vi "initialise.vi"(8 "error in (no error)":errorcluster, 11 "DL090623TwoDAnalyser in":refnum<class "AnalyserDL090623TwoD.lvclass">) -> (0 "error out":errorcluster, 3 "DL090623TwoDAnalyser out":refnum<class "AnalyserDL090623TwoD.lvclass">)   [LabVIEW 2010, in "AnalyserDL090623TwoD.lvclass"]
doc: "The dynamic dispatch-version of this VI initalises the plug-in object by allocating and initalising any dynamic resources need."
uses:
  AnalyserDL090623TwoD.lvclass
  common/classes/Image/Image/Image.lvclass
  AnalyserDL090624Scaffold/AnalyserDL090624Scaffold/AnalyserDL090624Scaffold.lvclass
  Segmenter/GenericSegmenter/GenericSegmenter/GenericSegmenter.lvclass
  TraceProcessor/GenericTraceProcessor/GenericTraceProcessor/GenericTraceProcessor.lvclass
  common/classes/ErrorController/ErrorController/ErrorController.lvclass
  common/enumerations/top-level_component_type_enum.ctl
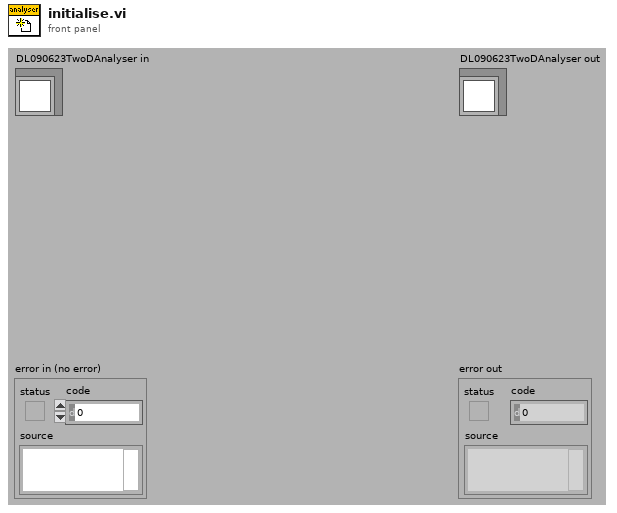
[diagram p1: front panel]
types:
  T1 = typedef "top-level_component_type_enum.ctl" = enum16{"undefined", "ImagingMode", "ScanHead", "DAQ", "ImageAssembler", "Display", "DataCollection", "Analyser", "Stimulator", "ExperimentController", "Instrument", "Stage"}
  T2 = typedef "Image Type" = u32
  T3 = typedef "plugin_specification.ctl" = cluster{"class path":string, "configuration":string, "label":string, "settings name":string}
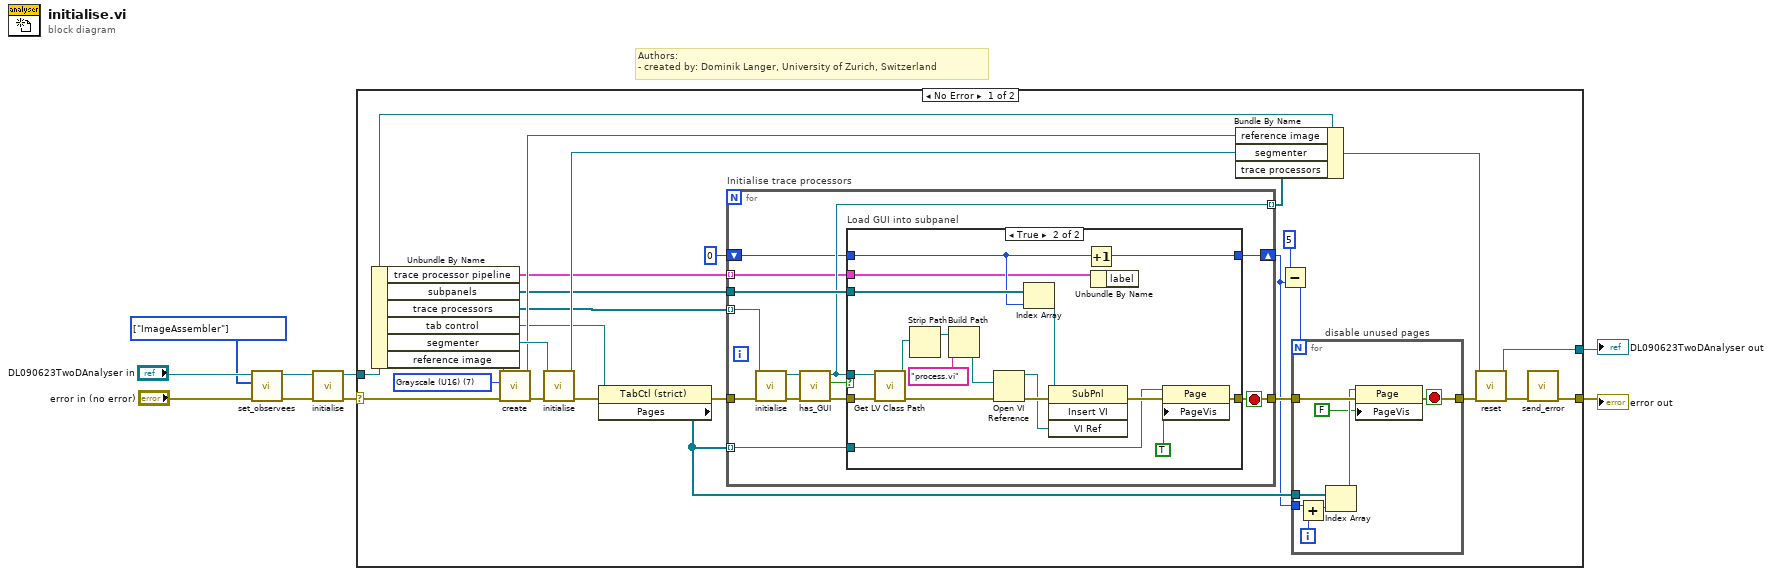
[diagram p0: block diagram]
diagram:
  w1 = T1[] [enum."ImageAssembler"] items=["undefined", "ImagingMode", "ScanHead", "DAQ", "ImageAssembler", "Display", "DataCollection", "Analyser", "Stimulator", "ExperimentController", "Instrument", "Stage"] ("observees")
  # "Authors: \n- created by: Dominik Langer, University of Zurich, Switzerland"
  n1 = call-dynamic "set_observees.vi"("error in (no error)"="error in (no error)", "observees"=w1, "GenericToplevelComponent in"="DL090623TwoDAnalyser in") -> ("error out"=w2:errorcluster, "GenericToplevelComponent out"=w4:refnum<class "AnalyserDL090623TwoD.lvclass">)  [unwired: 7 in]
  n2 = call-parent "initialise.vi"("error in (no error)"=w2, "GenericPlugin in"=w4) -> ("error out"=w9:errorcluster, "GenericPlugin out"=w8:refnum<class "AnalyserDL090623TwoD.lvclass">)  [unwired: 8 out]
  n3 = case shown="No Error" w9 {
    selector: w9 -> [w10 w78]
    tunnel: w8 -> [w11 w77]
    tunnel: [w12 w78] -> w7
    tunnel: [w32 w77] -> w6
    frame No Error {
      w34 = T2 7 items=["Grayscale (U8)", "Grayscale (I16)", "Grayscale (SGL)", "Complex (CSG)", "RGB (U32)", "HSL (U32)", "RGB (U64)", "Grayscale (U16)"] ("Image Type")
      n4 = Unbundle By Name(w11) -> ("trace processor pipeline"=w20:T3[], "subpanels"=w25:refnum<vi>[], "trace processors"=w27:refnum<class "GenericTraceProcessor.lvclass">[], "tab control"=w21:refnum<vi>, "segmenter"=w31:refnum<class "GenericSegmenter.lvclass">, "reference image"=w35:refnum<class "Image.lvclass">)
      n5 = call "create.vi"("error in (no error)"=w10, "Image Type"=w34, "Image in"=w35) -> ("error out"=w30:errorcluster, "Image out"=w28:refnum<class "Image.lvclass">)  [unwired: 1 in, 6 out]
      n6 = call-dynamic "initialise.vi"("error in (no error)"=w30, "GenericPlugin in"=w31) -> ("error out"=w23:errorcluster, "GenericPlugin out"=w29:refnum<class "GenericSegmenter.lvclass">)  [unwired: 8 out]
      n7 = property class="TabCtl (strict)"(reference=w21, error in=w23) -> (error out=w22:errorcluster, "Pages"=w17:refnum<vi>[])  [unwired: 1 out]
      n8 = for "Initialise trace processors" {
        tunnel: w27 -> [w55] mode=indexing
        tunnel: [w49] -> w26 mode=indexing
        tunnel: w25 -> [w51]
        shift-right: [w47] -> w16
        shift-left: 0 -> [w48]
        tunnel: w17 -> [w46] mode=indexing
        tunnel: w20 -> [w45] mode=indexing
        tunnel: w22 -> [w56]
        tunnel: [w44] -> w19
        stop <- w44 stop-if-true
        n9 = call-dynamic "initialise.vi"("error in (no error)"=w56, "GenericPlugin in"=w55) -> ("error out"=w54:errorcluster, "GenericPlugin out"=w53:refnum<class "GenericTraceProcessor.lvclass">)  [unwired: 8 out]
        n10 = call-dynamic "has_GUI.vi"("error in (no error)"=w54, "GenericTraceProcessor in"=w53) -> ("error out"=w52:errorcluster, "has GUI?"=w50:bool, "GenericTraceProcessor out"=w49:refnum<class "GenericTraceProcessor.lvclass">)  [unwired: 7 out]
        n11 = case "Load GUI into subpanel" shown="True" w50 {
          tunnel: w52 -> [w58 w72]
          tunnel: [w58 w62] -> w44
          tunnel: w51 -> [_ w76]
          tunnel: w49 -> [_ w70]
          tunnel: w48 -> [w57 w64]
          tunnel: [w57 w65] -> w47
          tunnel: w46 -> [_ w61]
          tunnel: w45 -> [_ w60]
          frame False {
          }
          frame True {
            n12 = call <vilib>:"Get LV Class Path.vi"("error in (no error)"=w72, "object"=w70) -> ("error out"=w71:errorcluster, "class path"=w69:path)  [unwired: 8 out]
            n13 = Strip Path(path=w69) -> (stripped path=w68:path)  [unwired: 1 out]
            n14 = Build Path(base path=w68, name or relative path="process.vi") -> (appended path=w66:path)
            n15 = Open VI Reference(vi path=w66, error in (no error)=w71) -> (vi reference=w73:refnum<vi>, error out=w74:errorcluster)  [unwired: 4 out]
            n16 = Index Array(array=w76, index=w64) -> (element=w75:refnum<vi>)
            n17 = invoke on="Invoke Node" class="SubPnl" method="Insert VI"(reference=w75, error in=w74, "VI Ref"=w73) -> (error out=w63:errorcluster)  [unwired: 1 in, 3 out]
            n18 = Increment(x=w64) -> (x+1=w65:i32)
            n19 = Unbundle By Name(w60) -> ()  [unwired: 1 out]
            n20 = property class="Page"(reference=w61, error in=w63, "PageVis"=TRUE) -> (error out=w62:errorcluster)  [unwired: 1 out]
          }
        }
      }
      n21 = Bundle By Name(cluster=w11, "reference image"=w28, "segmenter"=w29, "trace processors"=w26) -> (w33:refnum<class "AnalyserDL090623TwoD.lvclass">)
      n22 = Subtract(x=5, y=w16) -> (x-y=w15:i32)
      n23 = for "disable unused pages" {
        N: w15 -> [_]
        tunnel: w17 -> [w43]
        tunnel: w16 -> [w38]
        tunnel: w19 -> [w42]
        tunnel: [w36] -> w18
        i -> [w39]
        stop <- w36 stop-if-true
        n24 = Add(x=w38, y=w39) -> (x+y=w37:i32)
        n25 = Index Array(array=w43, index=w37) -> (element=w41:refnum<vi>)
        n26 = property class="Page"(reference=w41, error in=w42, "PageVis"=FALSE ("Page Visible")) -> (error out=w36:errorcluster)  [unwired: 1 out]
      }
      n27 = call-dynamic "reset.vi"("error in (no error)"=w18, "DL090623TwoDAnalyser in"=w33) -> ("error out"=w13:errorcluster, "DL090623TwoDAnalyser out"=w32:refnum<class "AnalyserDL090623TwoD.lvclass">)  [unwired: 8 out]
      n28 = call "send_error.vi"("error in (no error)"=w13) -> ("error out"=w12:errorcluster)  [unwired: 10 in]
    }
    frame Error {
    }
  }
  "error out" <- w7
  "DL090623TwoDAnalyser out" <- w6
